vi "_Get Mass Limits.vi"() -> (1 "Max":dbl, 2 "Min":dbl)   [LabVIEW 2012]
uses:
  _Global Configuration.vi
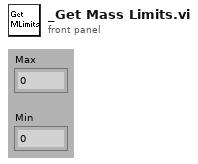
[diagram p1: front panel]
types:
  T1 = typedef "_RT Instrument 2.ctl" = cluster{"Table":T2[], "Instrument":string[]}
  T2 = typedef "_RT Configuration 2.ctl" = cluster{"Name":string, "Ch#":u8, "Min":dbl, "Max":dbl, "Def+":dbl, "Def-":dbl, "Offset":dbl, "Slope":dbl, "Type":u8, "Description":string, "SettleT":dbl}
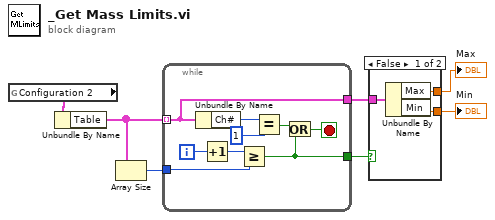
[diagram p0: block diagram]
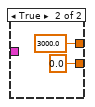
[diagram p2: hidden frame]
diagram:
  n1 = global read "_Global Configuration.vi" "Configuration 2"() -> (w5:T1)
  n2 = Unbundle By Name(w5) -> ("Table"=w4:T2[])
  n3 = Array Size(array=w4) -> (size(s)=w3:i32)
  n4 = while {
    tunnel: w4 -> [w14] mode=indexing
    tunnel: w3 -> [w11]
    tunnel: [w14] -> w2
    tunnel: [w8] -> w1
    i -> [w12]
    stop <- w9 stop-if-true
    n5 = Unbundle By Name(w14) -> ("Ch#"=w16:u8)
    n6 = Increment(x=w12) -> (x+1=w10:i32)
    n7 = Greater Or Equal?(x=w10, y=w11) -> (x >= y?=w8:bool)
    n8 = Equal?(x=w16, y=u8 1) -> (x = y?=w13:bool)
    n9 = Or(x=w13, y=w8) -> (x .or. y?=w9:bool)
  }
  n10 = case shown="False" w1 {
    tunnel: [w19 0.0 ("Min")] -> w7
    tunnel: [w18 3000.0 ("Max")] -> w6
    tunnel: w2 -> [w17 _]
    frame False {
      n11 = Unbundle By Name(w17) -> ("Max"=w18:dbl, "Min"=w19:dbl)
    }
    frame True {
    }
  }
  "Min" <- w7
  "Max" <- w6
